vi "UnoLoopbackTesterv3.vi"() -> ()   [LabVIEW 2009]
uses:
  <vilib>/Instr/_visa.llb/VISA Configure Serial Port (Instr).vi
panel:
  in  "stop":bool
  in  "System":enum32{"Main", "Serial Terminal"}(tab)=enum."Serial Terminal"
  out "Outgoing Messages":string
  in  "Send":bool
  in  "Input":string
  out "Incoming Messages":string
  in  "VISA resource name":refnum<visa-resource-name>
  in  "baud rate (9600)":u32=9600
  in  "data bits (8)":u16=8 min=5 max=8 step=1
  in  "parity (0:none)":enum16{"None", "Odd", "Even", "Mark", "Space"}(ring)
  in  "stop bits (10: 1 bit)":u16(ring)=10 items=["1.0"=10, "1.5"=15, "2.0"=20]
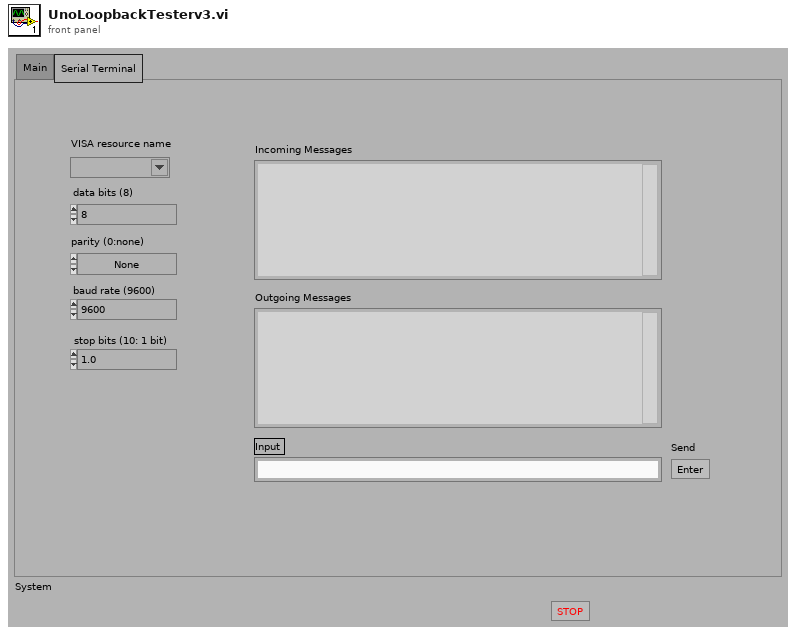
[diagram p1: front panel]
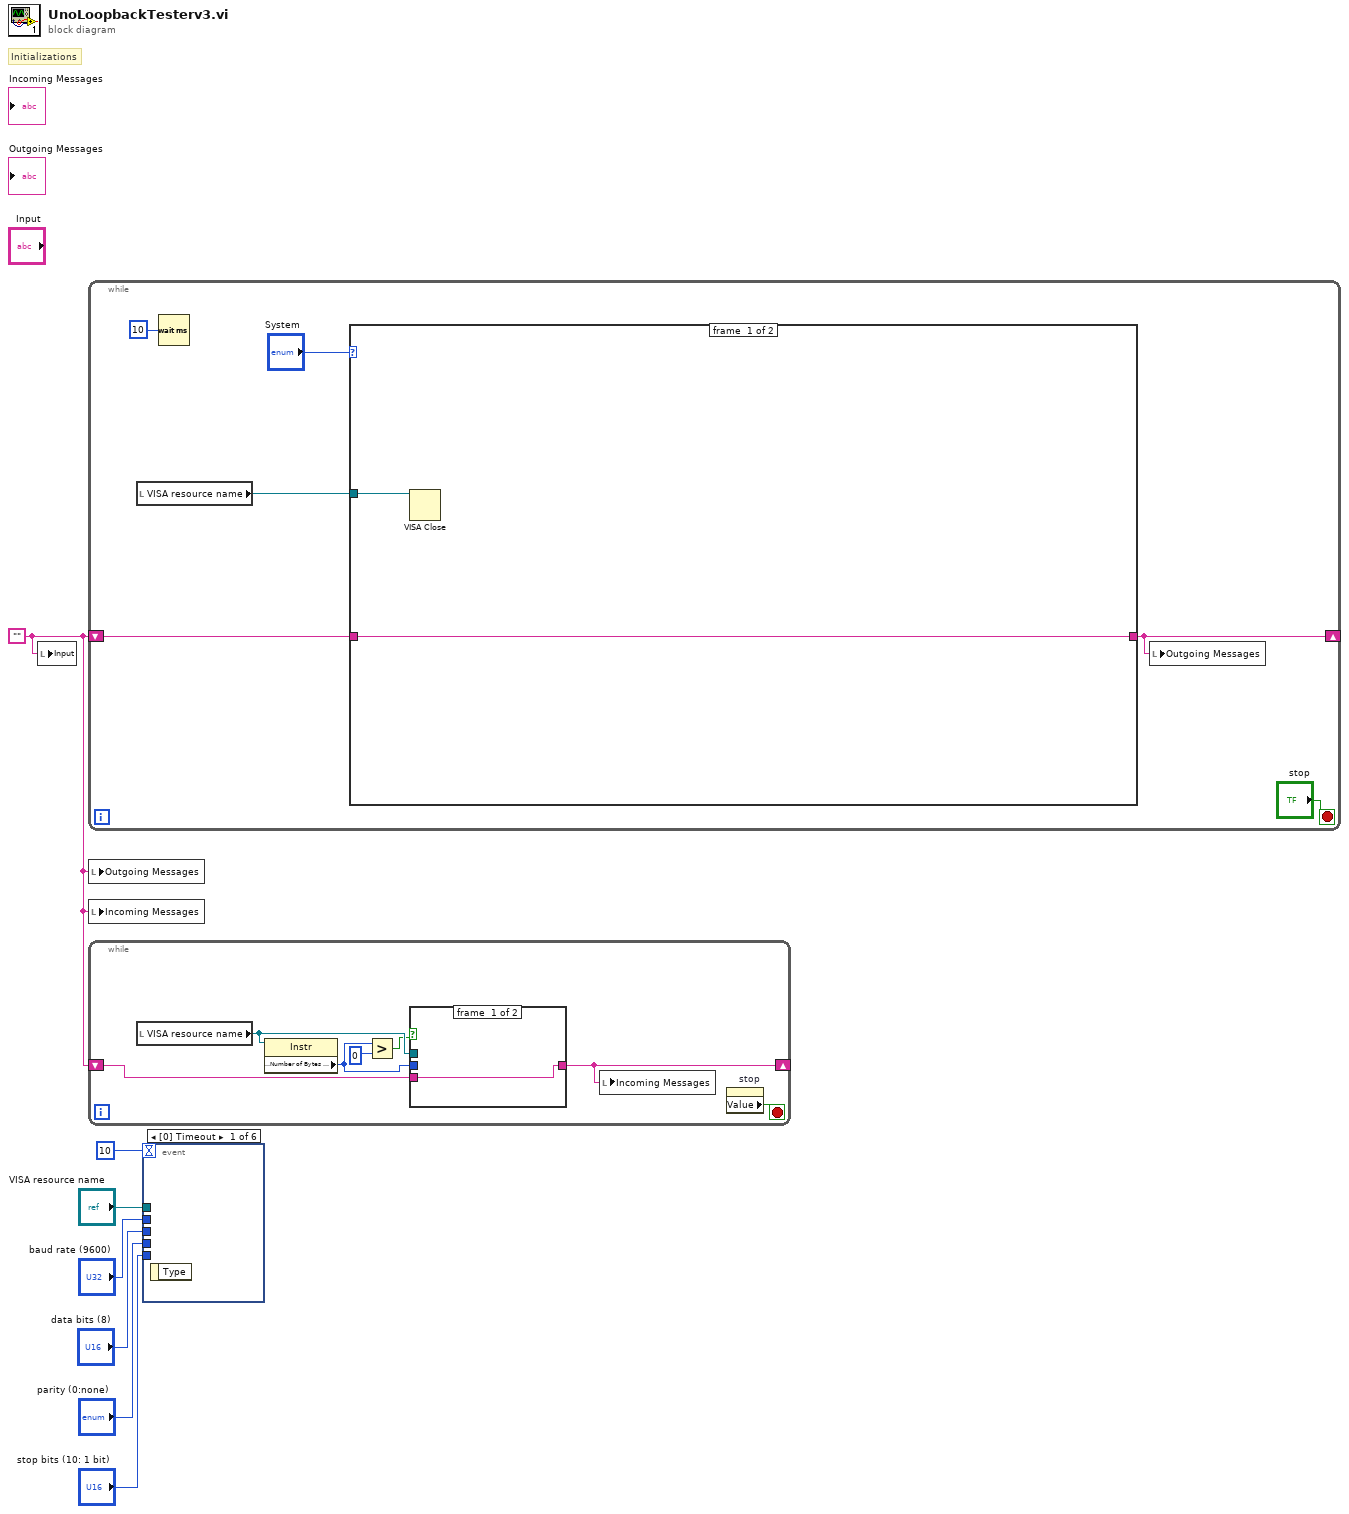
[diagram p0: block diagram]
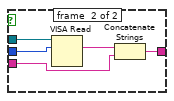
[diagram p2: hidden frame]
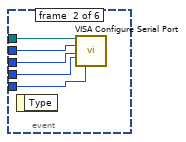
[diagram p3: hidden frame]
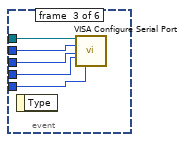
[diagram p4: hidden frame]
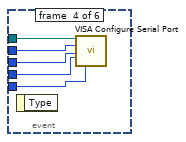
[diagram p5: hidden frame]
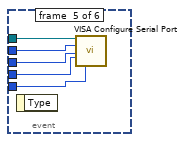
[diagram p6: hidden frame]
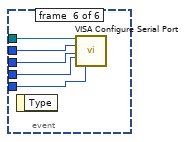
[diagram p7: hidden frame]
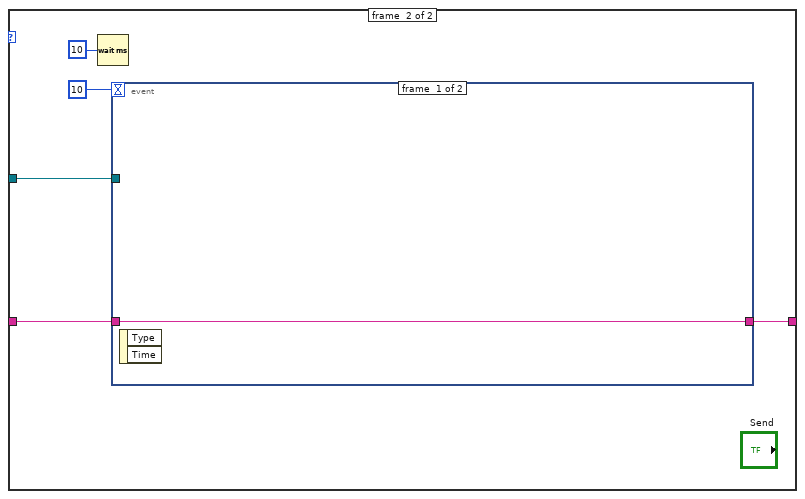
[diagram p8: hidden frame]
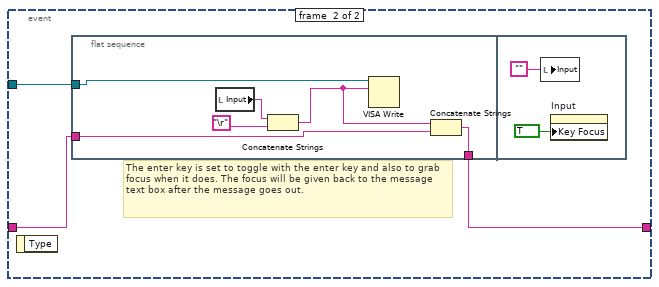
[diagram p9: hidden frame]
diagram:
  w1 = ""
  # "Initializations"
  n1 = local write "Input"(w1) -> ()
  n2 = while {
    shift-right: [w9] -> _
    shift-left: w1 -> [w10]
    stop <- "stop" stop-if-true
    n3 = local read "VISA resource name"() -> (w11:refnum<visa-resource-name>)
    n4 = Wait (ms)(milliseconds to wait=u32 10) -> ()  [unwired: 1 out]
    n5 = case shown="\"Serial Terminal\"" "System" {
      tunnel: w11 -> [w15 w18]
      tunnel: [w14 w17] -> w9
      tunnel: w10 -> [w14 w16]
      frame #0 {
        n6 = VISA Close(VISA resource name=w15) -> ()  [unwired: 1 in, 1 out]
      }
      frame #1 {
        n7 = Wait (ms)(milliseconds to wait=u32 10) -> ()  [unwired: 1 out]
        n8 = event shown="[1] \"Send\": Value Change" {
          selector: _ -> [_ _]
          dyn-events: _ -> [_ _]
          timeout: 10 -> [_ _]
          tunnel: w18 -> [_ w24]
          tunnel: [w21 w22] -> w17
          tunnel: w16 -> [w21 w23]
          event #0 {
            n9 = event-data() -> ()  [unwired: 1 in, 2 out]
          }
          event #1 {
            # "The enter key is set to toggle with the enter key and also to grab focus when it does. The focus will be given back to the message text box after the message goes out."
            n10 = event-data() -> ()  [unwired: 1 in, 1 out]
            n11 = flat-sequence {
              tunnel: w24 -> [w28]
              tunnel: w23 -> [w26]
              tunnel: [w25] -> w22
              frame #0 {
                n12 = local read "Input"() -> (w30:string)
                n13 = Concatenate Strings(w30, "\r") -> (w27:string)
                n14 = VISA Write(VISA resource name=w28, write buffer=w27) -> ()  [unwired: 1 in, 3 out]
                n15 = Concatenate Strings(w27, w26) -> (w25:string)
              }
              frame #1 {
                n16 = local write "Input"("") -> ()
                n17 = property on="Input" class="Str"("Key Focus"=TRUE) -> ()  [unwired: 2 in, 2 out]
              }
            }
          }
        }
      }
    }
    n18 = local write "Outgoing Messages"(w9) -> ()
  }
  n19 = local write "Outgoing Messages"(w1) -> ()
  n20 = local write "Incoming Messages"(w1) -> ()
  n21 = while {
    shift-right: [w33] -> _
    shift-left: w1 -> [w34]
    stop <- w38 stop-if-true
    n22 = local read "VISA resource name"() -> (w39:refnum<visa-resource-name>)
    n23 = property class="Instr"(reference=w39) -> ("Serial Settings:Number of Bytes at Serial Port"=w35:u32)  [unwired: 1 in, 2 out]
    n24 = Greater?(x=w35, y=u32 0) -> (0:w36:bool)
    n25 = case shown="True" w36 {
      tunnel: w39 -> [_ w45]
      tunnel: w35 -> [_ w44]
      tunnel: w34 -> [w40 w41]
      tunnel: [w40 w42] -> w33
      frame #0 {
      }
      frame #1 {
        n26 = VISA Read(VISA resource name=w45, byte count=w44) -> (read buffer=w43:string)  [unwired: 1 in, 3 out]
        n27 = Concatenate Strings(w43, w41) -> (w42:string)
      }
    }
    n28 = local write "Incoming Messages"(w33) -> ()
    n29 = property on="stop" class="Bool (strict)"() -> ("Value"=w38:bool)  [unwired: 2 in, 2 out]
  }
  n30 = event shown="[0] Timeout" {
    selector: _ -> [_ _ _ _ _ _]
    dyn-events: _ -> [_ _ _ _ _ _]
    timeout: 10 -> [_ _ _ _ _ _]
    tunnel: "VISA resource name" -> [_ w50 w55 w60 w65 w70]
    tunnel: "baud rate (9600)" -> [_ w49 w54 w59 w64 w69]
    tunnel: "data bits (8)" -> [_ w48 w53 w58 w63 w68]
    tunnel: "parity (0:none)" -> [_ w47 w52 w57 w62 w67]
    tunnel: "stop bits (10: 1 bit)" -> [_ w46 w51 w56 w61 w66]
    event #0 {
      n31 = event-data() -> ()  [unwired: 1 in, 1 out]
    }
    event #1 {
      n32 = event-data() -> ()  [unwired: 1 in, 1 out]
      n33 = call-poly "VISA Configure Serial Port"("VISA resource name"=w50, "baud rate (9600)"=w49, "data bits (8)"=w48, "parity (0:none)"=w47, "stop bits (10: 1 bit)"=w46) -> ()  [unwired: 9 in, 2 out]
    }
    event #2 {
      n34 = event-data() -> ()  [unwired: 1 in, 1 out]
      n35 = call-poly "VISA Configure Serial Port"("VISA resource name"=w55, "baud rate (9600)"=w54, "data bits (8)"=w53, "parity (0:none)"=w52, "stop bits (10: 1 bit)"=w51) -> ()  [unwired: 9 in, 2 out]
    }
    event #3 {
      n36 = event-data() -> ()  [unwired: 1 in, 1 out]
      n37 = call-poly "VISA Configure Serial Port"("VISA resource name"=w60, "baud rate (9600)"=w59, "data bits (8)"=w58, "parity (0:none)"=w57, "stop bits (10: 1 bit)"=w56) -> ()  [unwired: 9 in, 2 out]
    }
    event #4 {
      n38 = event-data() -> ()  [unwired: 1 in, 1 out]
      n39 = call-poly "VISA Configure Serial Port"("VISA resource name"=w65, "baud rate (9600)"=w64, "data bits (8)"=w63, "parity (0:none)"=w62, "stop bits (10: 1 bit)"=w61) -> ()  [unwired: 9 in, 2 out]
    }
    event #5 {
      n40 = event-data() -> ()  [unwired: 1 in, 1 out]
      n41 = call-poly "VISA Configure Serial Port"("VISA resource name"=w70, "baud rate (9600)"=w69, "data bits (8)"=w68, "parity (0:none)"=w67, "stop bits (10: 1 bit)"=w66) -> ()  [unwired: 9 in, 2 out]
    }
  }
